vi "WF_control.vi"(0 "Start V":dbl format="%#_13g", 1 "Step V":dbl format="%#_13g", 2 "End V":dbl format="%#_13g", 3 "Ramp Time (ms)":u32, 4 "COM Keithley":refnum<visa-resource-name>, 5 "COM WF":refnum<visa-resource-name>, 6 "ERR Keithley":errorcluster, 7 "ERR WF":errorcluster) -> (8 "XY图":cluster{dbl[], dbl[]}(graph))   [LabVIEW 2018]
uses:
  <instrlib>/Keithley 648X Series/Keithley 648X Series.lvlib
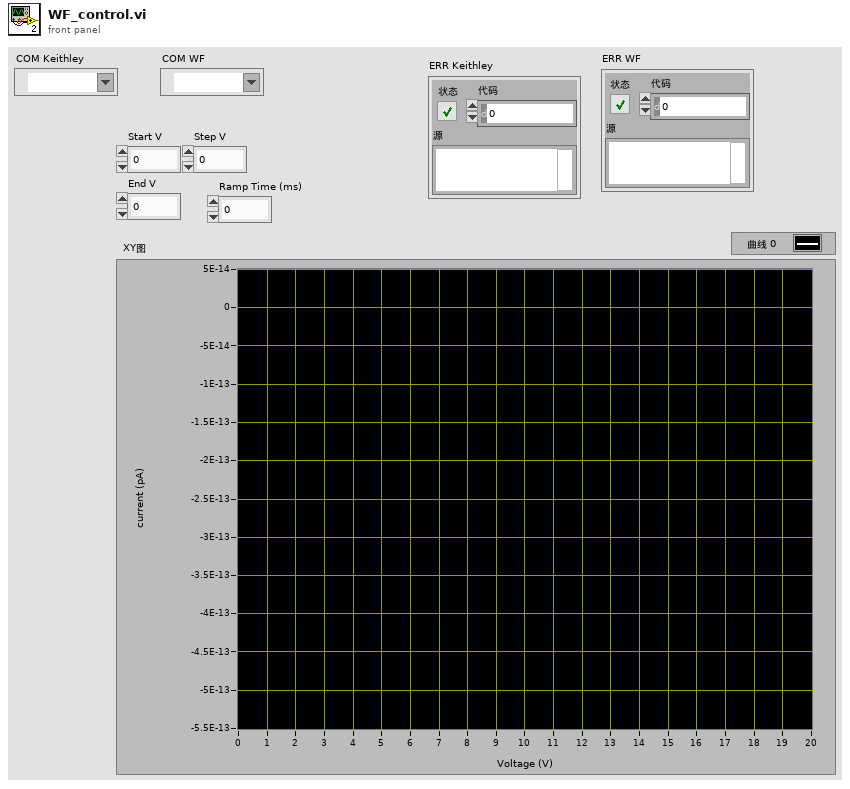
[diagram p1: front panel]
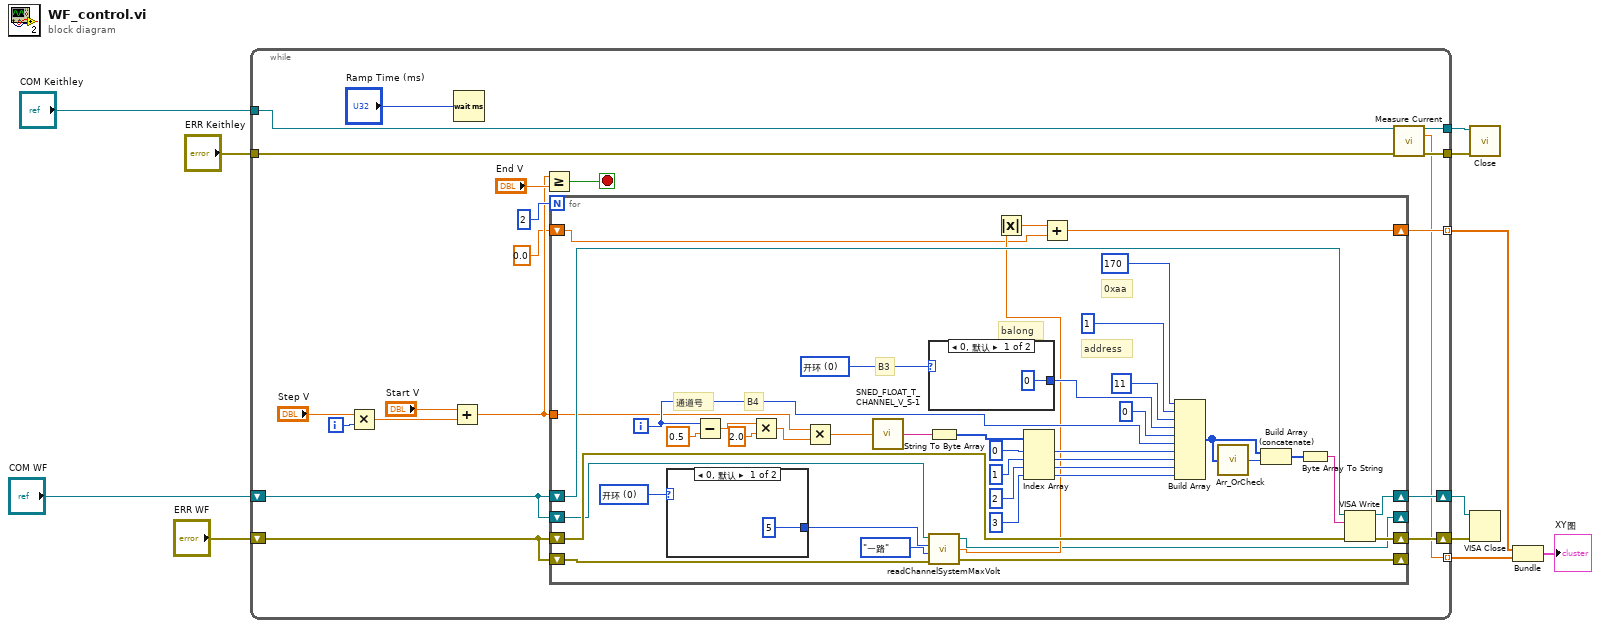
[diagram p0: block diagram]
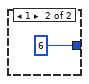
[diagram p2: hidden frame]
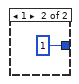
[diagram p3: hidden frame]
diagram:
  n1 = while {
    shift-right: [w31] -> w9
    shift-left: "COM WF" -> [w20]
    shift-right: [w30] -> w8
    shift-left: "ERR WF" -> [w19]
    tunnel: [w12] -> w7 mode=indexing
    tunnel: [w17] -> w5 mode=indexing
    tunnel: "COM Keithley" -> [w16]
    tunnel: "ERR Keithley" -> [w15]
    tunnel: [w14] -> w4
    tunnel: [w13] -> w3
    i -> [w28]
    stop <- w26 stop-if-true
    n2 = Multiply(x="Step V", y=w28) -> (x*y=w27:dbl)
    n3 = Add(x="Start V", y=w27) -> (x+y=w21:dbl)
    n4 = Wait (ms)(milliseconds to wait="Ramp Time (ms)") -> ()  [unwired: 1 out]
    n5 = Greater Or Equal?(x=w21, y="End V") -> (x >= y?=w26:bool)
    n6 = for {
      N: 2 -> [_]
      shift-right: [w71] -> w31
      shift-left: w20 -> [w73]
      shift-right: [w70] -> w30
      shift-left: w19 -> [w72]
      tunnel: w21 -> [w41]
      shift-right: [w36] -> _
      shift-left: w20 -> [w38]
      shift-right: [w35] -> _
      shift-left: w19 -> [w37]
      shift-right: [w32] -> w17
      shift-left: 0.0 -> [w33]
      i -> [w46]
      w48 = u16 0 items=["  开环", "  闭环"] ("开闭环")
      w51 = u16 0 items=["  开环", "  闭环"] ("开闭环")
      # "通道号"
      # "B4"
      # "B3"
      # "balong"
      # "address"
      # "0xaa"
      n7 = case shown="0, 默认" w48 {
        tunnel: [5 6] -> w49
        frame 0, Default {
        }
        frame 1 {
        }
      }
      n8 = Subtract(x=w46, y=0.5) -> (x-y=w44:dbl)
      n9 = Multiply(x=w44, y=2.0) -> (x*y=w42:dbl)
      n10 = Multiply(x=w41, y=w42) -> (x*y=w40:dbl)
      n11 = call "SNED_FLOAT_T_CHANNEL_V_S-1.vi"("数据"=w40) -> ("字符串"=w69:string)
      n12 = case shown="0, 默认" w51 {
        tunnel: [0 1] -> w58
        frame 0, Default {
        }
        frame 1 {
        }
      }
      n13 = String To Byte Array(string=w69) -> (unsigned byte array=w68:u8[])
      n14 = call "readChannelSystemMaxVolt.vi"("error out 2"=w37, "通道号"=enum16{"一路", "二路", "三路"}."一路" ("通道选择"), "B3"=w49, "VISA resource name out 2"=w38) -> ("error out"=w35:errorcluster, "输出变量"=w39:dbl, "VISA resource name out"=w36:refnum<visa-resource-name>)
      n15 = Absolute Value(x=w39) -> (abs(x)=w34:dbl)
      n16 = Index Array(array=w68, index #1=0, index #2=1, index #3=2, index #4=3) -> (element #1=w56:u8, element #2=w55:u8, element #3=w54:u8, element #4=w53:u8)
      n17 = Add(x=w34, y=w33) -> (x+y=w32:dbl)
      n18 = Build Array(170, 1, 11, w58, 0, w46, w56, w55, w54, w53) -> (w52:i32[])
      n19 = call "Arr_OrCheck.vi"("数组"=w52) -> ("抑或的数据值"=w63:u8)
      n20 = Build Array (concatenate)(w52, w63) -> (w62:i32[])
      n21 = Byte Array To String(unsigned byte array=w62) -> (string=w50:string)
      n22 = VISA Write(VISA resource name=w73, write buffer=w50, error in (no error)=w72) -> (VISA resource name out=w71:refnum<visa-resource-name>, error out=w70:errorcluster)  [unwired: 1 out]
    }
    n23 = call <instrlib>:"Measure Current.vi"("VISA resource name"=w16, "error in (no error)"=w15) -> ("VISA resource name out"=w14:refnum<visa-resource-name>, "Measurement"=w12:dbl, "error out"=w13:errorcluster)  [unwired: 11 in]
  }
  n24 = call <instrlib>:"Close.vi"("error in (no error)"=w3, "VISA resource name"=w4) -> ()  [unwired: 9 in, 1 out]
  n25 = VISA Close(VISA resource name=w9, error in (no error)=w8) -> ()  [unwired: 1 out]
  n26 = Bundle(w5, w7) -> (→"XY图":cluster{dbl[], dbl[]})  [unwired: 1 in]
